vi "Encode String.vi"(7 "Prepend BOM (F)":bool, 8 "error in":errorcluster, 9 "Output Encoding (UTF-16LE)":T1=enum."UTF-16LE", 10 "Input Encoding (ANSI)":T1, 11 "String in":string) -> (0 "error out":errorcluster, 3 "String out":string)   [LabVIEW 2020, in "G-Unicode.lvlib"]
doc: "Encodes the text in <b>String</b> with the encoding specified by <b>Output Encoding</b>. The input String encoding is defined by <b>Input Encoding</b>. If Output Encoding is unicode (UTF-8 or UTF-16), the corresponding Byte Order Mark (BOM) can be prepended by setting <b>Prepend BOM</b> to TRUE.\n\nIf the input string encoding isn't known, Input Encoding can be set to Auto to try and automatically detect the encoding method. Note that automatic encoding detection isn't 100% accurate, and it is recommended to set the encoding explicitly if it is known.\n\nSupported input/output encodings:\nANSI\nUTF-8\nUTF-16LE"
uses:
  G-Unicode.lvlib
  Controls/Input String Encoding.ctl
  Controls/String Encoding.ctl
  Private/Conversion/Polymorphic VIs/Text to UTF-8 (LabVIEW String).vi
  Private/Conversion/Polymorphic VIs/UTF-8 to Text (LabVIEW String).vi
  SubVIs/Byte Order Marks.vi
  Detect BOM.vi
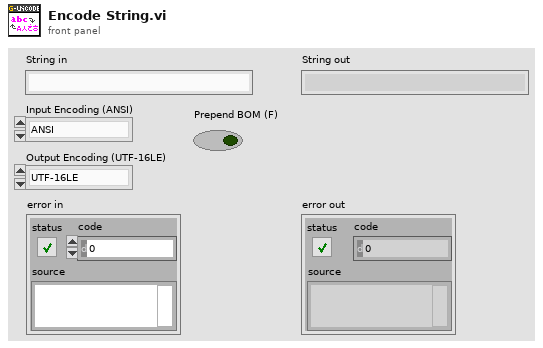
[diagram p1: front panel]
types:
  T1 = typedef "G-Unicode.lvlib/Input String Encoding.ctl" = enum16{"ANSI", "UTF-8", "UTF-16LE", "UTF-16BE", "Auto"}
  T2 = typedef "G-Unicode.lvlib/String Encoding.ctl" = enum16{"ANSI", "UTF-8", "UTF-16LE", "UTF-16BE", "Unknown"}
  T3 = typedef "G-Unicode.lvlib/Encoded UTF-8 String.ctl" = string
  T4 = typedef "G-Unicode.lvlib/Encoded UTF-16LE String.ctl" = string
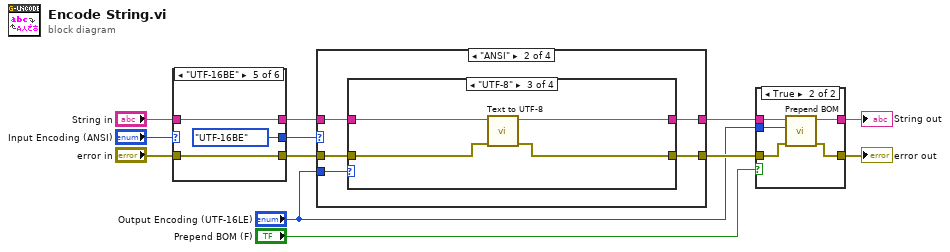
[diagram p0: block diagram]
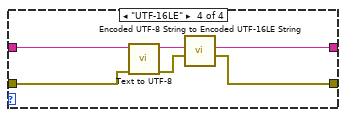
[diagram p6: hidden frame]
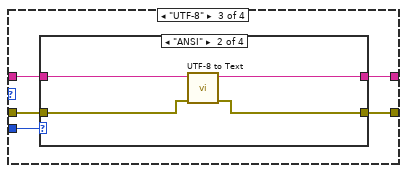
[diagram p7: hidden frame]
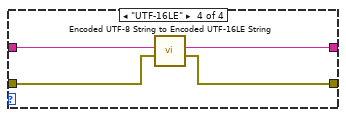
[diagram p10: hidden frame]
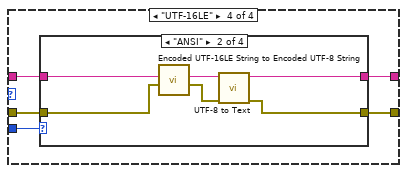
[diagram p11: hidden frame]
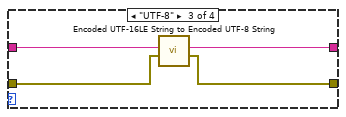
[diagram p13: hidden frame]
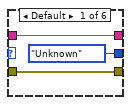
[diagram p15: hidden frame]
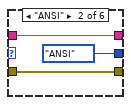
[diagram p16: hidden frame]
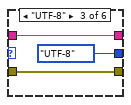
[diagram p17: hidden frame]
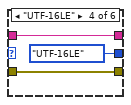
[diagram p18: hidden frame]
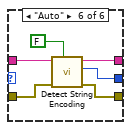
[diagram p19: hidden frame]
diagram:
  n1 = case shown="\"UTF-16BE\"" "Input Encoding (ANSI)" {
    tunnel: "String in" -> [w15 w17 w20 w23 w26 w33]
    tunnel: [String_Encoding."Unknown" ("Encoding") String_Encoding."ANSI" ("Encoding") String_Encoding."UTF-8" ("Encoding") String_Encoding."UTF-16LE" ("Encoding") String_Encoding."UTF-16BE" ("Encoding") w32] -> w8
    tunnel: [w15 w17 w20 w23 w26 w31] -> w9
    tunnel: "error in" -> [w13 w16 w19 w22 w25 w28]
    tunnel: [w13 w16 w19 w22 w25 w29] -> w7
    frame Default {
    }
    frame "ANSI" {
    }
    frame "UTF-8" {
    }
    frame "UTF-16LE" {
    }
    frame "UTF-16BE" {
    }
    frame "Auto" {
      n2 = call "Detect String Encoding.vi"("Strip BOM (T)"=FALSE ("Remove BOM (T)"), "error in"=w28, "String"=w33) -> ("error out"=w29:errorcluster, "Encoding"=w32:T2, "String out"=w31:string)  [unwired: 6 in]
    }
  }
  n3 = case shown="\"ANSI\"" w8 {
    tunnel: w9 -> [w35 w39 w57 w74]
    tunnel: "Output Encoding (UTF-16LE)" -> [_ w36 w59 w76]
    tunnel: w7 -> [w34 w38 w56 w73]
    tunnel: [w35 w40 w58 w75] -> w6
    tunnel: [w34 w37 w55 w72] -> w4
    frame Default {
    }
    frame "ANSI" {
      n4 = case shown="\"UTF-8\"" w36 {
        tunnel: [w42 w44 w45 w52] -> w40
        tunnel: w39 -> [w42 w44 w48 w54]
        tunnel: w38 -> [w41 w43 w47 w51]
        tunnel: [w41 w43 w46 w49] -> w37
        frame Default {
        }
        frame "ANSI" {
        }
        frame "UTF-8" {
          n5 = call-poly "Text to UTF-8.vi"("error in"=w47, "String"=w48) -> ("error out"=w46:errorcluster, "UTF-8 Encoded String"=w45:T3)  [unwired: 8 in]
        }
        frame "UTF-16LE" {
          n6 = call-poly "Text to UTF-8.vi"("error in"=w51, "String"=w54) -> ("error out"=w50:errorcluster, "UTF-8 Encoded String"=w53:T3)  [unwired: 8 in]
          n7 = call "Encoded UTF-8 String to Encoded UTF-16LE String.vi"("error in"=w50, "Encoded UTF-8 String"=w53) -> ("error out"=w49:errorcluster, "Encoded UTF-16LE String"=w52:T4)  [unwired: 8 in]
        }
      }
    }
    frame "UTF-8" {
      n8 = case shown="\"ANSI\"" w59 {
        tunnel: [w61 w64 w66 w71] -> w58
        tunnel: w57 -> [w61 w65 w66 w69]
        tunnel: w56 -> [w60 w62 w67 w68]
        tunnel: [w60 w63 w67 w70] -> w55
        frame Default {
        }
        frame "ANSI" {
          n9 = call-poly "UTF-8 to Text.vi"("error in"=w62, "UTF-8 Encoded String"=w65) -> ("error out"=w63:errorcluster, "String"=w64:string)  [unwired: 8 in]
        }
        frame "UTF-8" {
        }
        frame "UTF-16LE" {
          n10 = call "Encoded UTF-8 String to Encoded UTF-16LE String.vi"("error in"=w68, "Encoded UTF-8 String"=w69) -> ("error out"=w70:errorcluster, "Encoded UTF-16LE String"=w71:T4)  [unwired: 8 in]
        }
      }
    }
    frame "UTF-16LE" {
      n11 = case shown="\"ANSI\"" w76 {
        tunnel: [w78 w84 w88 w89] -> w75
        tunnel: w74 -> [w78 w81 w87 w89]
        tunnel: w73 -> [w77 w79 w85 w90]
        tunnel: [w77 w83 w86 w90] -> w72
        frame Default {
        }
        frame "ANSI" {
          n12 = call "Encoded UTF-16LE String to Encoded UTF-8 String.vi"("error in"=w79, "Encoded UTF-16LE String"=w81) -> ("error out"=w80:errorcluster, "Encoded UTF-8 String"=w82:T3)  [unwired: 8 in]
          n13 = call-poly "UTF-8 to Text.vi"("error in"=w80, "UTF-8 Encoded String"=w82) -> ("error out"=w83:errorcluster, "String"=w84:string)  [unwired: 8 in]
        }
        frame "UTF-8" {
          n14 = call "Encoded UTF-16LE String to Encoded UTF-8 String.vi"("error in"=w85, "Encoded UTF-16LE String"=w87) -> ("error out"=w86:errorcluster, "Encoded UTF-8 String"=w88:T3)  [unwired: 8 in]
        }
        frame "UTF-16LE" {
        }
      }
    }
  }
  n15 = case shown="True" "Prepend BOM (F)" {
    tunnel: w6 -> [w92 w97]
    tunnel: [w92 w96] -> w5
    tunnel: w4 -> [w91 w95]
    tunnel: [w91 w94] -> w3
    tunnel: "Output Encoding (UTF-16LE)" -> [_ w93]
    frame False {
    }
    frame True {
      n16 = call "Prepend BOM.vi"("error in"=w95, "Input Encoding (UTF-16LE)"=w93, "String"=w97) -> ("error out"=w94:errorcluster, "String with BOM"=w96:string)  [unwired: 7 in]
    }
  }
  "String out" <- w5
  "error out" <- w3
